vi "MathematicalOperators.vi"() -> ()   [LabVIEW 2020]
panel:
  in  "B":dbl
  in  "A":dbl
  out "A / B":dbl
  out "A * B":dbl
  out "A - B":dbl
  out "A+B":dbl
  # "Add, Multiply, Subtract and Divide two numeric inputs"
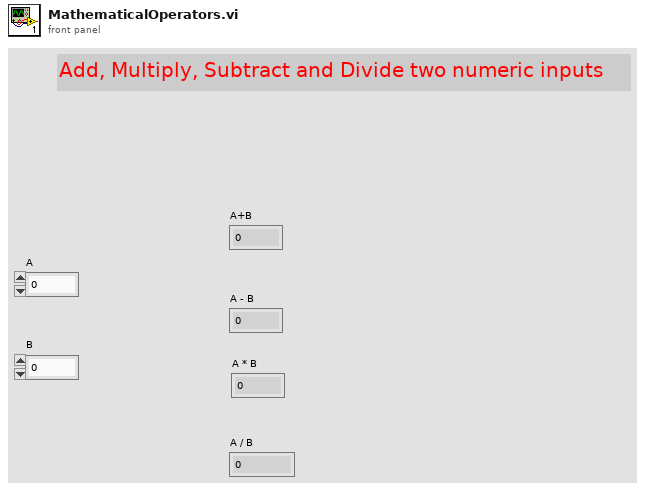
[diagram p1: front panel]
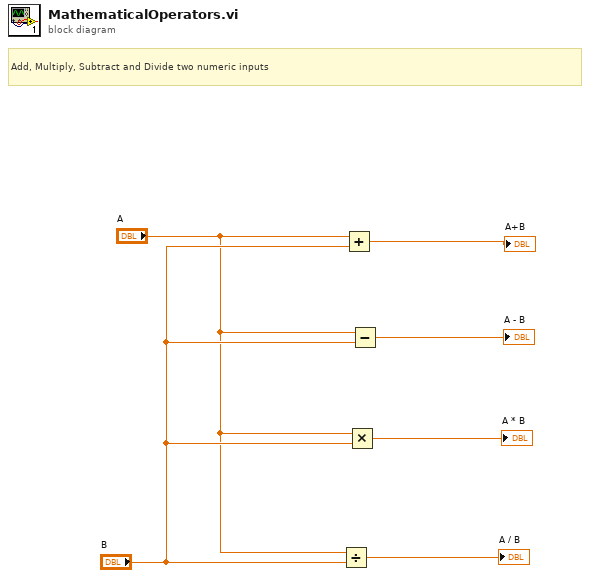
[diagram p0: block diagram]
diagram:
  # "Add, Multiply, Subtract and Divide two numeric inputs"
  n1 = Divide(x="A", y="B") -> (x/y=→"A / B":dbl)
  n2 = Add(x="A", y="B") -> (x+y=→"A+B":dbl)
  n3 = Multiply(x="A", y="B") -> (x*y=→"A * B":dbl)
  n4 = Subtract(x="A", y="B") -> (x-y=→"A - B":dbl)
